vi "EST Output Constructor.vi"(8 "error in (no error)":errorcluster, 9 "Project Item":cluster{"Name":string, "Value":variant}[](array[cluster]), 10 "Load Path":path, 11 "Memory Template Path":path) -> (0 "error out":errorcluster, 3 "EST Output.lvclass":refnum<class "EST Output.lvclass">)   [LabVIEW 2019, in "EST Output.lvclass"]
uses:
  EST Output.lvclass
  EST Output.lvclass/EST Output.ctl
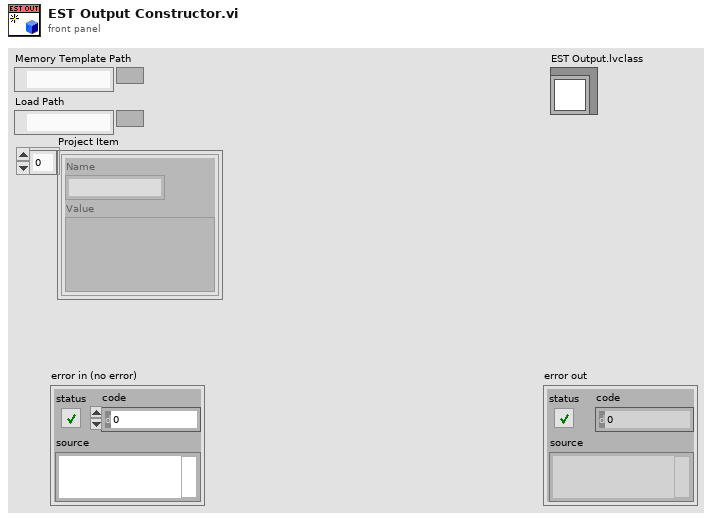
[diagram p1: front panel]
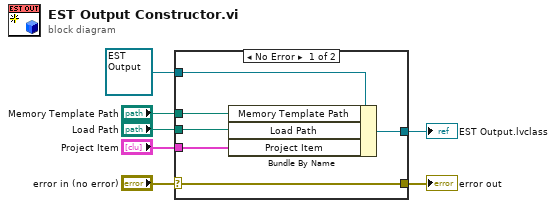
[diagram p0: block diagram]
diagram:
  n1 = case shown="No Error" "error in (no error)" {
    selector: "error in (no error)" -> [w8 w15]
    tunnel: refnum<class "EST Output.lvclass"> refnum ("EST Output.lvclass") -> [w13 w14]
    tunnel: [w12 w14] -> w6
    tunnel: "Memory Template Path" -> [w11 _]
    tunnel: "Load Path" -> [w10 _]
    tunnel: "Project Item" -> [w9 _]
    tunnel: [w8 w15] -> w1
    frame No Error {
      n2 = Bundle By Name(cluster=w13, "Memory Template Path"=w11, "Load Path"=w10, "Project Item"=w9) -> (w12:refnum<class "EST Output.lvclass">)
    }
    frame Error {
    }
  }
  "EST Output.lvclass" <- w6
  "error out" <- w1
